vi "Launch Digital Twin UI.vi"(8 "error in (no error)":errorcluster) -> (0 "error out":errorcluster)   [LabVIEW 2018, in "Digtial Twin.lvlib"]
uses:
  Digtial Twin.lvlib
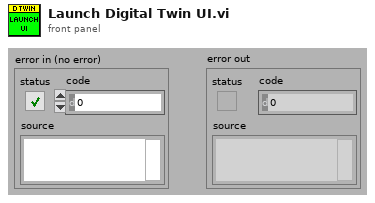
[diagram p1: front panel]
types:
  T1 = enum32{"Bad", "Idle", "Run top level", "Running"}
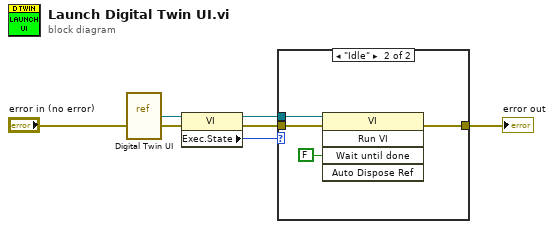
[diagram p0: block diagram]
diagram:
  n1 = vi-ref "Digital Twin UI.vi"() -> (w6:refnum<vi>)
  n2 = property class="VI"(reference=w6, error in="error in (no error)") -> (reference out=w2:refnum<vi>, error out=w3:errorcluster, "Exec.State"=w4:T1)
  n3 = case shown="\"Idle\"" w4 {
    tunnel: w3 -> [w7 w8]
    tunnel: w2 -> [_ w9]
    tunnel: [w7 w10] -> w1
    frame Default {
    }
    frame "Idle" {
      n4 = invoke class="VI" method="Run VI"(reference=w9, error in=w8, "Wait until done"=FALSE ("Wait Until Done")) -> (error out=w10:errorcluster)  [unwired: 2 in, 4 out]
    }
  }
  "error out" <- w1
